vi "qrread.vi"() -> ()   [LabVIEW 2019]
uses:
  Global 1.vi
  <vilib>/vision/driver/NI_Vision_Acquisition_Software.lvlib
  <vilib>/userDefined/High Color/IMAQdx.ctl
  <vilib>/myRIO/Instrument Drivers/Utilities/Utilities.lvlib
  <vilib>/myRIO/Common/Instrument Driver Framework/myRIO v1.0/DIO/typedefs/DIO Channels Enum.ctl
  <vilib>/myRIO/Common/Instrument Driver Framework/myRIO v1.0/DIO/typedefs/DIO Channels List.ctl
  <vilib>/myRIO/Common/Instrument Driver Framework/Utilities/typedefs/Generic FPGA Reference.ctl
  <vilib>/myRIO/Common/Instrument Driver Framework/Utilities/typedefs/myRIO v1.0 Reference.ctl
  <vilib>/myRIO/Common/Instrument Driver Framework/Utilities/typedefs/Hardware Version Enum.ctl
  <vilib>/myRIO/Common/Instrument Driver Framework/Utilities/typedefs/myRIO Generic Hardware Reference.ctl
  <vilib>/myRIO/Instrument Drivers/Onboard IO/DIO/typedefs/DIO Reference.ctl
  <vilib>/myRIO/Instrument Drivers/Onboard IO/DIO/DIO.lvlib
  <vilib>/myRIO/Instrument Drivers/Onboard IO/DIO/vis/Write.vi
  <vilib>/userDefined/High Color/nirio_resource_hc.ctl
  <vilib>/myRIO/Common/Instrument Driver Framework/myRIO v1.0/DIO/vis/myRIO v1.1 Open DIO.vi
  <vilib>/myRIO/Instrument Drivers/Onboard IO/DIO/vis/myRIO DIO Open.xnode
  <vilib>/myRIO/Common/Instrument Driver Framework/Utilities/vis/Is FPGA Ref Available.vi
  <vilib>/myRIO/Express VI/Onboard Devices/LED/LED Express VI.xnode
  <vilib>/myRIO/Express VI/Onboard IO/DO/DO Express VI.xnode
  <vilib>/myRIO/Express VI/Onboard IO/DI/DI Express VI.xnode
  <vilib>/myRIO/Instrument Drivers/Onboard IO/DIO/vis/Read.vi
  <vilib>/vision/Instrument.llb/QR Code Model Type.ctl
  <vilib>/vision/Instrument.llb/QR Code Stream Mode Type.ctl
  <vilib>/vision/Instrument.llb/Data Matrix Polarity.ctl
  <vilib>/vision/Instrument.llb/Demodulation Mode.ctl
  <vilib>/vision/Instrument.llb/Cell Sample Size.ctl
  <vilib>/vision/Instrument.llb/Cell Filter Mode.ctl
  <vilib>/vision/Instrument.llb/QR Code Report.ctl
panel:
  out "Refnum out 4":T1(plugin-control)
  out "Refnum out 3":T1(plugin-control)
  in  "Error/Flow In":errorcluster
  out "Refnum out 2":T1(plugin-control)
  out "Refnum out":T1(plugin-control)
  out "t":i32
  out "Array":bool[](array[boolean])
  out "appended array":bool[](array[boolean])
  out "Found?":bool
  out "Bounding Box":cluster{"x":sgl, "y":sgl}[](array[cluster])
  out "QR Barcode Report (2D Barcode Reader 1)":T2={"Found?"=FALSE, "Data"="", "Bounding Box"=[], "Errors Corrected"=0, "Dimensions (Rows/Cols)"=0, "Version"=0, "QR Model"=3, "Stream Mode"=0, "Barcode Polarity"=-2, "Mirrored?"=FALSE, "Append Stream Position"=0, "Size of Append Stream"=0, "First EAN-128 ID"=0, "First Alternate Language ID"=0, "Append Stream ID"=0, "Minimum Edge Strength"=30, "Demodulation Mode"=-2, "Cell Sample Size"=-2, "Cell Filter Mode"=-2} {"Append Stream ID" format="%x"; "Cell Filter Mode" items=["Auto-detect"=-2, "Average"=0, "Median"=1, "Central Average"=2, "High Average"=3, "Low Average"=4, "Very High Average"=5, "Very Low Average"=6, "All Filters"=8]; "Cell Sample Size" items=["Auto-detect"=-2, "1x1"=1, "2x2"=2, "3x3"=3, "4x4"=4, "5x5"=5, "6x6"=6, "7x7"=7]; "Demodulation Mode" items=["Auto-detect"=-2, "Histogram"=0, "Local Contrast"=1, "Combination"=2, "All"=3]; "Barcode Polarity" items=["Auto-detect"=-2, "Black on White"=0, "White on Black"=1]; "Stream Mode" items=["Auto-detect", "Numeric", "AlphaNumeric", "Mixed", "Raw Bytes", "UCC/EAN-128 - In Tokens", "UCC/EAN-128 - In Data", "Extended Character Interpretation", "Kanji"]; "QR Model" items=["Auto Detect", "Micro", "Model 1", "Model 2"]; "Version" max=40 step=1}
  in  "Stop (F)":bool
  out "Image Out":T1(plugin-control)
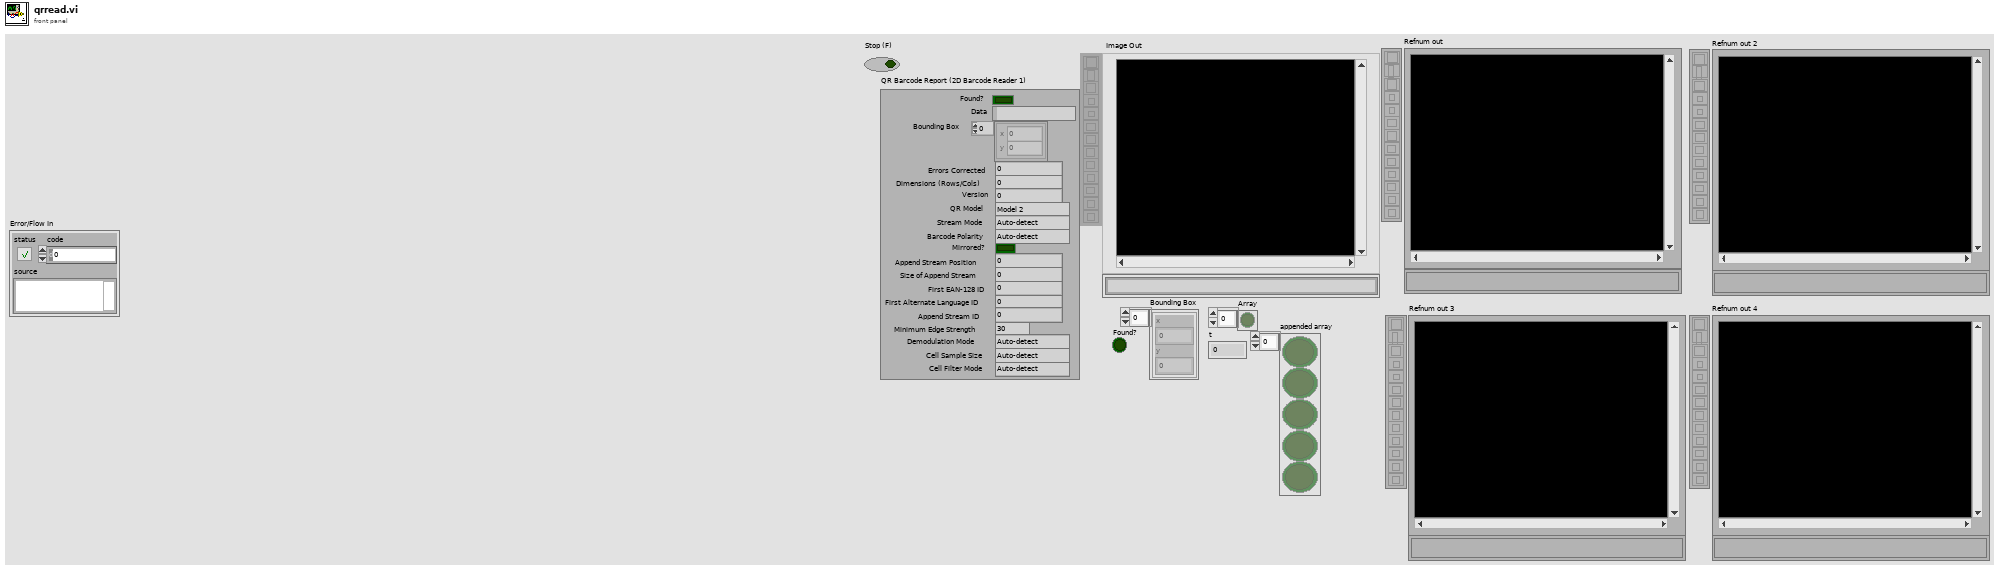
[diagram p1: front panel]
types:
  T1 = typedef "IMAQ Image.ctl" = refnum<image>
  T2 = typedef "QR Code Report.ctl" = cluster{"Found?":bool, "Data":string, "Bounding Box":cluster{"x":sgl, "y":sgl}[], "Errors Corrected":u32, "Dimensions (Rows/Cols)":u32, "Version":u32, "QR Model":T3, "Stream Mode":T4, "Barcode Polarity":T5, "Mirrored?":bool, "Append Stream Position":u32, "Size of Append Stream":u32, "First EAN-128 ID":i32, "First Alternate Language ID":i32, "Append Stream ID":u32, "Minimum Edge Strength":u32, "Demodulation Mode":T6, "Cell Sample Size":T7, "Cell Filter Mode":T8}
  T3 = typedef "QR Code Model Type.ctl" = i32
  T4 = typedef "QR Code Stream Mode Type.ctl" = i32
  T5 = typedef "Data Matrix Polarity.ctl" = i32
  T6 = typedef "Demodulation Mode.ctl" = i32
  T7 = typedef "Cell Sample Size.ctl" = i32
  T8 = typedef "Cell Filter Mode.ctl" = i32
  T9 = typedef "IMAQdx.ctl" = refnum<k21>
  T10 = typedef "DIO.lvlib/DIO Reference.ctl" = cluster{"myRIO Reference":T11, "DIO Channels List":T15}
  T11 = typedef "myRIO Generic Hardware Reference.ctl" = cluster{"myRIO Model":T12, "myRIO Hardware Reference":T13}
  T12 = typedef "Hardware Version Enum.ctl" = enum16{"Unknown", "myRIO-1900", "myRIO-1950", "roboRIO", "NI ELVIS RIO CM", "ELVIS III"}
  T13 = typedef "myRIO v1.0 Reference.ctl" = cluster{"Generic FPGA Reference":T14, "Allow multiple opens":bool}
  T14 = typedef "Generic FPGA Reference.ctl" = refnum<k20>
  T15 = typedef "DIO Channels List.ctl" = T16[]
  T16 = typedef "DIO Channels Enum.ctl" = enum16{"Not Connected", "C/DIO0", "C/DIO1", "C/DIO2", "C/DIO3", "C/DIO4", "C/DIO5", "C/DIO6", "C/DIO7", "A/DIO0", "A/DIO1", "A/DIO2", "A/DIO3", "A/DIO4", "A/DIO5", "A/DIO6", "A/DIO7", "A/DIO8", "A/DIO9", "A/DIO10", "A/DIO11", "A/DIO12", "A/DIO13", "A/DIO14", "A/DIO15", "A/DIO16", "A/DIO17", "A/DIO18", "A/DIO19", "B/DIO0", "B/DIO1", "B/DIO2", "B/DIO3", "B/DIO4", "B/DIO5", "B/DIO6", "B/DIO7", "B/DIO8", "B/DIO9", "B/DIO10", "B/DIO11", "B/DIO12", "B/DIO13", "B/DIO14", "B/DIO15", "B/DIO16", "B/DIO17", "B/DIO18", "B/DIO19", "LED0", "LED1", "LED2", "LED3", "Button0", "DIO/DIO0", "DIO/DIO1", "DIO/DIO2", "DIO/DIO3", "DIO/DIO4", "DIO/DIO5", "DIO/DIO6", "DIO/DIO7", "DIO/DIO8", "DIO/DIO9", "SPI/CS0", "SPI/CS1", "SPI/CS2", "SPI/CS3", "LED RADIO (Green)", "LED RADIO (Red)", "LED COMM (Green)", "LED COMM (Red)", "LED MODE (Green)", "LED MODE (Red)"}
  T17 = typedef "nirio_resource_hc.ctl" = tag
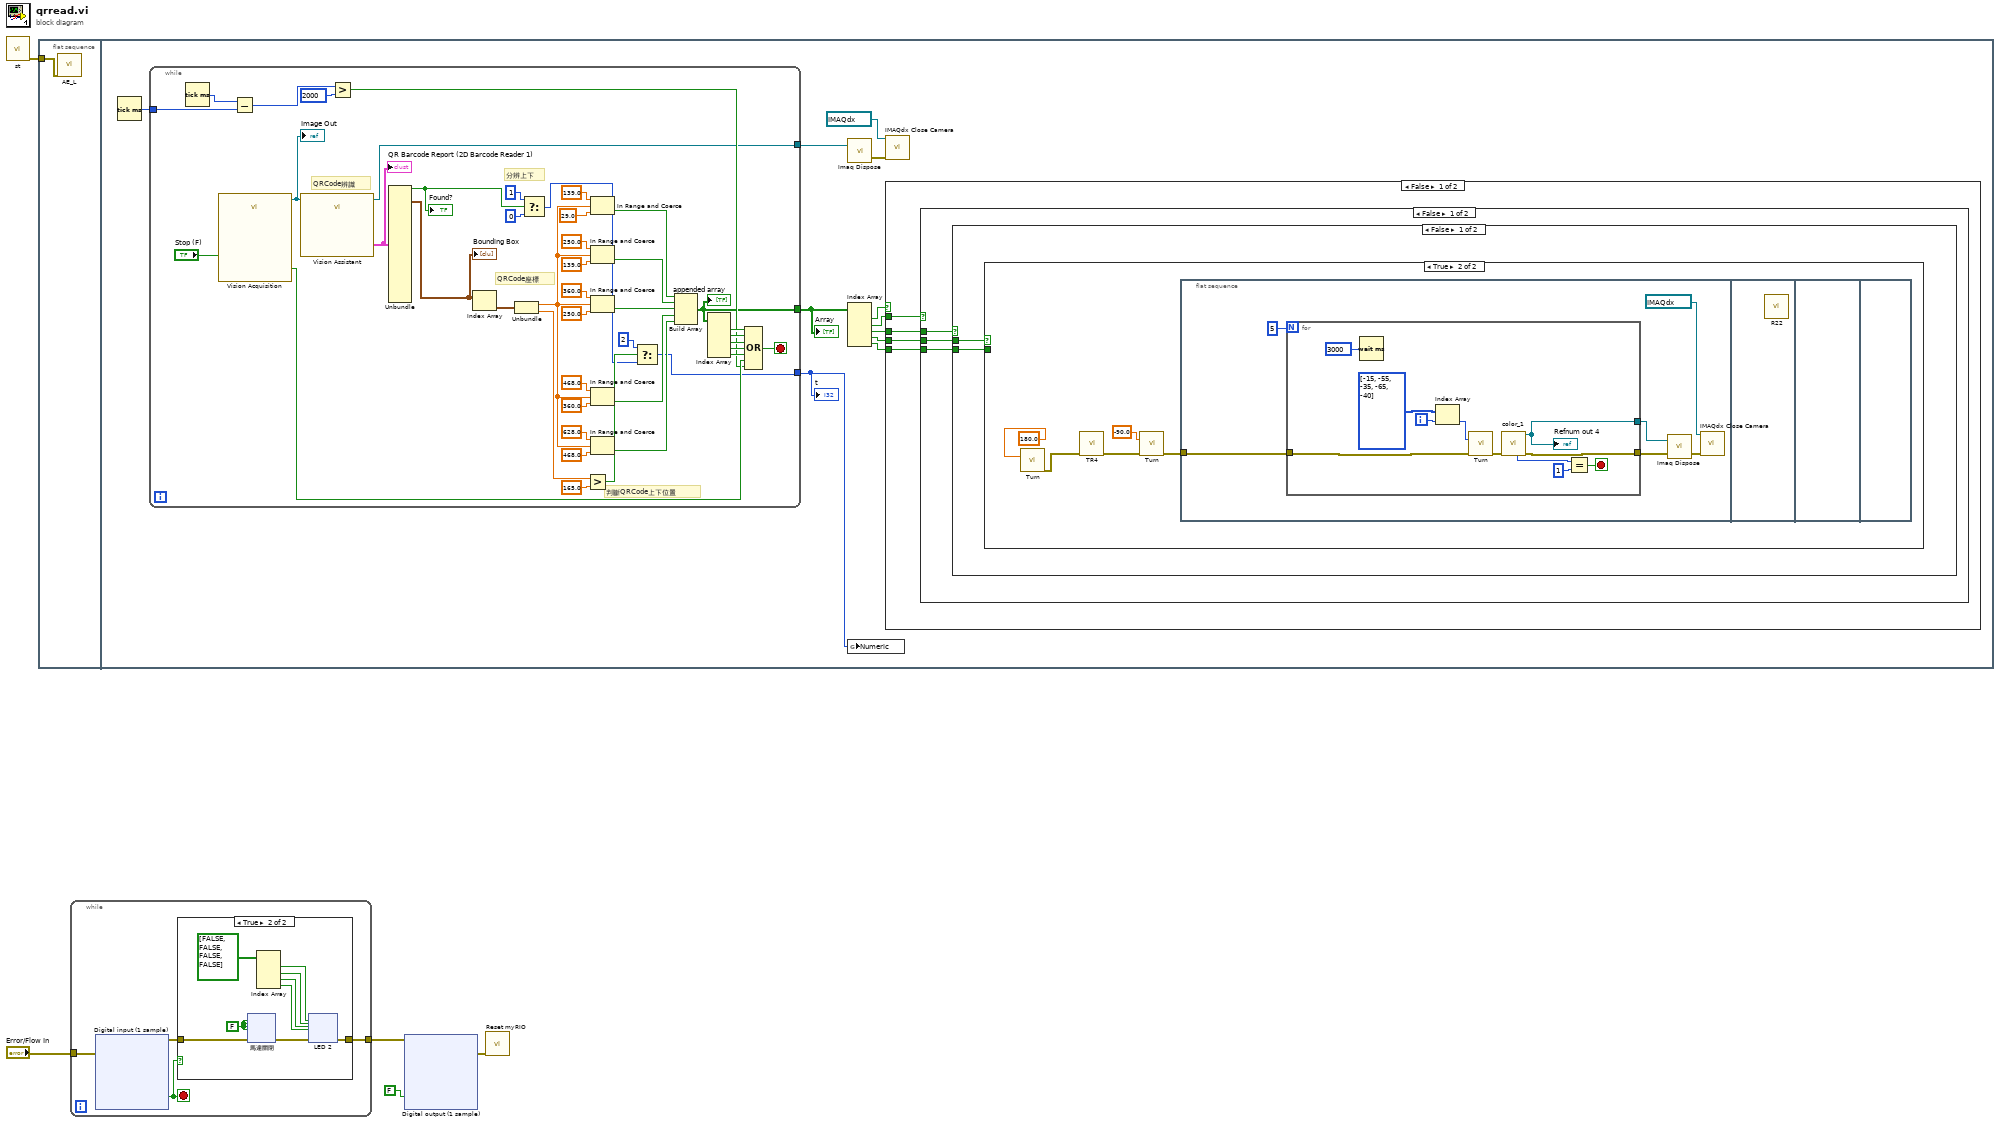
[diagram p0: block diagram]
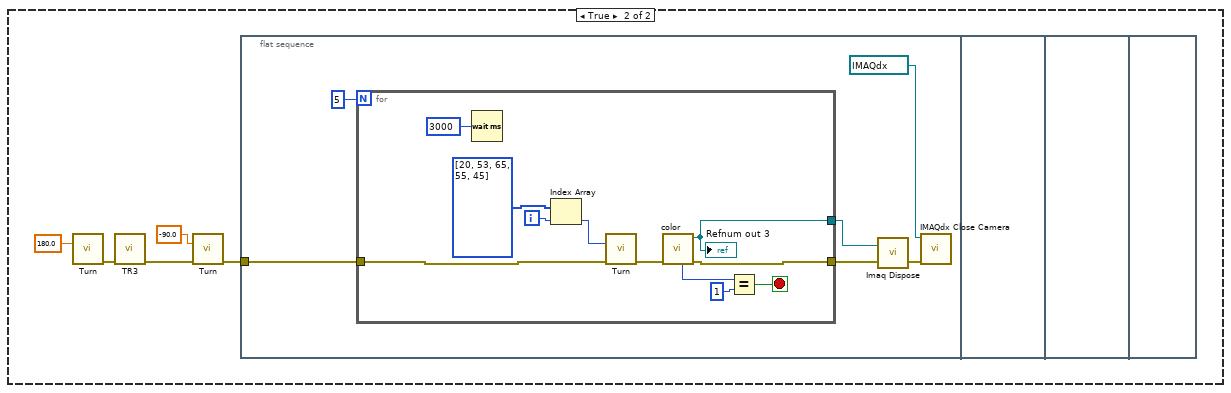
[diagram p5: hidden frame]
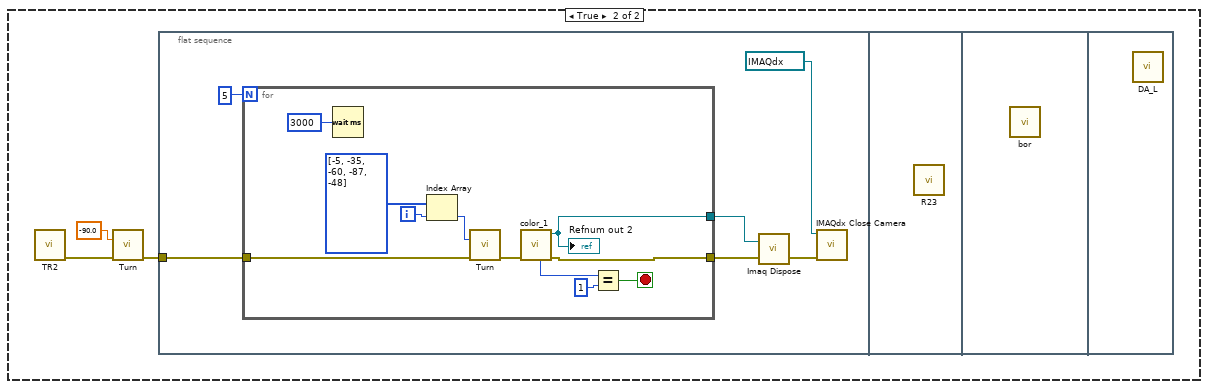
[diagram p6: hidden frame]
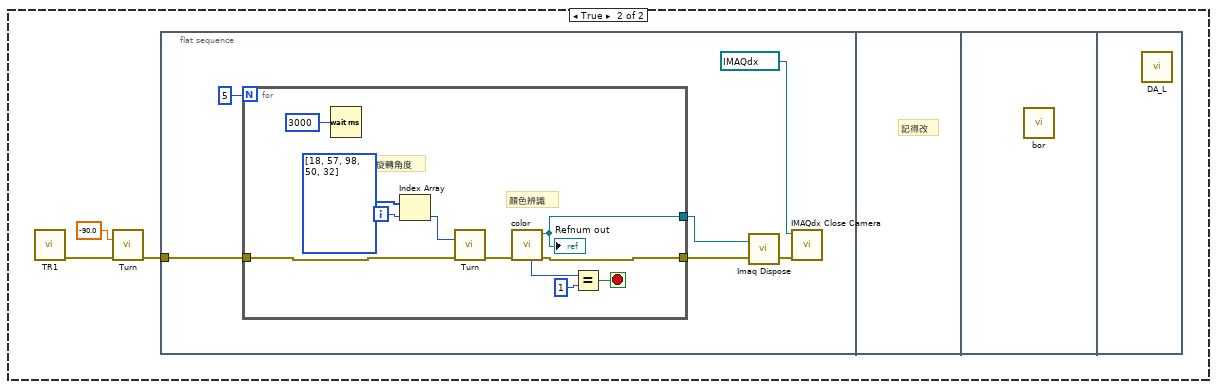
[diagram p7: hidden frame]
diagram:
  n1 = call "st.vi"() -> ("Error/Flow Out"=w5:errorcluster)  [unwired: 11 in]
  n2 = flat-sequence {
    tunnel: w5 -> [w6]
    frame #0 {
      n3 = call "AE_L.vi"("error in (no error)"=w6) -> ()  [unwired: 10 in, 1 out]
    }
    frame #1 {
      n4 = Tick Count (ms)() -> (millisecond timer value=w17:u32)
      n5 = while {
        tunnel: w17 -> [w135]
        tunnel: [w124] -> w16
        tunnel: [w115] -> w10
        tunnel: [w112] -> w9
        stop <- w125 stop-if-true
        # "分辨上下"
        # "QRCode辨識"
        # "判斷QRCode上下位置"
        # "QRCode座標"
        n6 = Tick Count (ms)() -> (millisecond timer value=w136:u32)
        n7 = call "Vision Acquisition"("Stop (F)"="Stop (F)") -> ("Image Out"=w114:T1, "Stopped"=w127:bool)  [unwired: 24 in, 1 out]
        "Image Out" <- w114
        n8 = Subtract(x=w136, y=w135) -> (x-y=w134:u32)
        n9 = call "Vision Assistant"("Image In"=w114) -> ("Image Out"=w112:T1, "QR Barcode Report (2D Barcode Reader 1)"=w113:T2)  [unwired: 24 in, 1 out]
        "QR Barcode Report (2D Barcode Reader 1)" <- w113
        n10 = Greater?(x=w134, y=u32 2000) -> (0:w126:bool)
        n11 = Unbundle(w113) -> ("Found?"=w120:bool, "Bounding Box"=w154:cluster{"x":sgl, "y":sgl}[])  [unwired: 17 out]
        "Bounding Box" <- w154
        "Found?" <- w120
        n12 = Index Array(array=w154) -> (element=w143:cluster{"x":sgl, "y":sgl})  [unwired: 1 in]
        n13 = Unbundle(w143) -> ("x"=w142:sgl, "y"=w123:sgl)
        n14 = Select(t=1, s=w120, f=0) -> (s? t:f=w117:i32)
        n15 = Greater?(x=w123, y=sgl 165.0) -> (0:w121:bool)
        n16 = In Range and Coerce(upper limit=139.0, x=w142, lower limit=29.0) -> (In Range?=w141:bool)  [unwired: 1 out]
        n17 = In Range and Coerce(upper limit=250.0, x=w142, lower limit=139.0) -> (In Range?=w140:bool)  [unwired: 1 out]
        n18 = In Range and Coerce(upper limit=360.0, x=w142, lower limit=250.0) -> (In Range?=w139:bool)  [unwired: 1 out]
        n19 = In Range and Coerce(upper limit=468.0, x=w142, lower limit=360.0) -> (In Range?=w138:bool)  [unwired: 1 out]
        n20 = In Range and Coerce(upper limit=628.0, x=w142, lower limit=468.0) -> (In Range?=w137:bool)  [unwired: 1 out]
        n21 = Select(t=2, s=w121, f=w117) -> (s? t:f=w115:i32)
        n22 = Build Array(w141, w140, w139, w138, w137) -> (w124:bool[])
        "appended array" <- w124
        n23 = Index Array(array=w124) -> (element #1=w132:bool, element #2=w131:bool, element #3=w130:bool, element #4=w129:bool, element #5=w128:bool)  [unwired: 5 in]
        n24 = Compound Arithmetic op=OR(w132, w131, w130, w129, w128, w127, w126) -> (w125:bool)
      }
      "Array" <- w16
      "t" <- w10
      n25 = call "Imaq Dispose"("Image"=w9) -> ("error out"=w8:errorcluster)  [unwired: 5 in]
      n26 = Index Array(array=w16) -> (element #1=w15:bool, element #2=w14:bool, element #3=w13:bool, element #4=w12:bool, element #5=w11:bool)  [unwired: 5 in]
      n27 = global write "Global 1.vi" "Numeric"(w10) -> ()
      n28 = call <vilib>:"IMAQdx Close Camera.vi"("error in"=w8, "Session In"=T9 "cam0") -> ()  [unwired: 9 in, 1 out]
      n29 = case shown="False" w15 {
        tunnel: w14 -> [w21 _]
        tunnel: w13 -> [w20 _]
        tunnel: w12 -> [w19 _]
        tunnel: w11 -> [w18 _]
        frame False {
          n30 = case shown="False" w21 {
            tunnel: w20 -> [w24 _]
            tunnel: w19 -> [w23 _]
            tunnel: w18 -> [w22 _]
            frame False {
              n31 = case shown="False" w24 {
                tunnel: w23 -> [w26 _]
                tunnel: w22 -> [w25 _]
                frame False {
                  n32 = case shown="True" w26 {
                    tunnel: w25 -> [w27 _]
                    frame False {
                      n33 = case shown="True" w27 {
                        frame False {
                        }
                        frame True {
                        }
                      }
                    }
                    frame True {
                      n34 = call "Turn.vi"("角度"=180.0) -> ("error out"=w28:errorcluster)  [unwired: 14 in]
                      n35 = call "TR4.vi"("error in (no error)"=w28) -> ("error out"=w29:errorcluster)  [unwired: 10 in]
                      n36 = call "Turn.vi"("角度"=-90.0, "error in (no error)"=w29) -> ("error out"=w31:errorcluster)  [unwired: 13 in]
                      n37 = flat-sequence {
                        tunnel: w31 -> [w37]
                        frame #0 {
                          n38 = for {
                            N: 5 -> [_]
                            tunnel: w37 -> [w42]
                            tunnel: [w40] -> w33
                            tunnel: [w39] -> w35
                            i -> [w45]
                            stop <- w46 stop-if-true
                            n39 = Wait (ms)(milliseconds to wait=u32 3000) -> ()  [unwired: 1 out]
                            n40 = Index Array(array=i32[] [-15, -55, -35, -65, -40], index=w45) -> (element=w44:i32)
                            n41 = call "Turn.vi"("角度"=w44, "error in (no error)"=w42) -> ("error out"=w41:errorcluster)  [unwired: 13 in]
                            n42 = call "color_1.vi"("error in"=w41) -> ("error out"=w40:errorcluster, "Refnum out"=w39:T1, "yellow"=w43:i32)  [unwired: 3 in, 5 out]
                            "Refnum out 4" <- w39
                            n43 = Equal?(x=w43, y=1) -> (x = y?=w46:bool)
                          }
                          n44 = call "Imaq Dispose"("Image"=w35, "error in (no error)"=w33) -> ("error out"=w34:errorcluster)  [unwired: 4 in]
                          n45 = call <vilib>:"IMAQdx Close Camera.vi"("error in"=w34, "Session In"=T9 "cam0") -> ()  [unwired: 9 in, 1 out]
                        }
                        frame #1 {
                          n46 = call "R22.vi"() -> ()  [unwired: 12 in]
                        }
                        frame #2 {
                        }
                        frame #3 {
                        }
                      }
                    }
                  }
                }
                frame True {
                  n47 = call "Turn.vi"("角度"=180.0) -> ("error out"=w54:errorcluster)  [unwired: 14 in]
                  n48 = call "TR3.vi"("error in (no error) 2"=w54) -> ("error out 2"=w50:errorcluster)  [unwired: 10 in]
                  n49 = call "Turn.vi"("角度"=-90.0, "error in (no error)"=w50) -> ("error out"=w52:errorcluster)  [unwired: 13 in]
                  n50 = flat-sequence {
                    tunnel: w52 -> [w59]
                    frame #0 {
                      n51 = for {
                        N: 5 -> [_]
                        tunnel: w59 -> [w65]
                        tunnel: [w63] -> w55
                        tunnel: [w61] -> w57
                        i -> [w67]
                        stop <- w68 stop-if-true
                        n52 = Wait (ms)(milliseconds to wait=u32 3000) -> ()  [unwired: 1 out]
                        n53 = Index Array(array=i32[] [20, 53, 65, 55, 45], index=w67) -> (element=w66:i32)
                        n54 = call "Turn.vi"("角度"=w66, "error in (no error)"=w65) -> ("error out"=w64:errorcluster)  [unwired: 13 in]
                        n55 = call "color.vi"("error in"=w64) -> ("error out"=w63:errorcluster, "Refnum out"=w61:T1, "yellow"=w62:i32)  [unwired: 3 in, 5 out]
                        "Refnum out 3" <- w61
                        n56 = Equal?(x=w62, y=1) -> (x = y?=w68:bool)
                      }
                      n57 = call "Imaq Dispose"("Image"=w57, "error in (no error)"=w55) -> ("error out"=w56:errorcluster)  [unwired: 4 in]
                      n58 = call <vilib>:"IMAQdx Close Camera.vi"("error in"=w56, "Session In"=T9 "cam0") -> ()  [unwired: 9 in, 1 out]
                    }
                    frame #1 {
                    }
                    frame #2 {
                    }
                    frame #3 {
                    }
                  }
                }
              }
            }
            frame True {
              n59 = call "TR2.vi"() -> ("error out"=w73:errorcluster)  [unwired: 11 in]
              n60 = call "Turn.vi"("角度"=-90.0, "error in (no error)"=w73) -> ("error out"=w74:errorcluster)  [unwired: 13 in]
              n61 = flat-sequence {
                tunnel: w74 -> [w79]
                frame #0 {
                  n62 = for {
                    N: 5 -> [_]
                    tunnel: w79 -> [w84]
                    tunnel: [w82] -> w75
                    tunnel: [w81] -> w77
                    i -> [w87]
                    stop <- w88 stop-if-true
                    n63 = Wait (ms)(milliseconds to wait=u32 3000) -> ()  [unwired: 1 out]
                    n64 = Index Array(array=i32[] [-5, -35, -60, -87, -48], index=w87) -> (element=w86:i32)
                    n65 = call "Turn.vi"("角度"=w86, "error in (no error)"=w84) -> ("error out"=w83:errorcluster)  [unwired: 13 in]
                    n66 = call "color_1.vi"("error in"=w83) -> ("error out"=w82:errorcluster, "Refnum out"=w81:T1, "yellow"=w85:i32)  [unwired: 3 in, 5 out]
                    "Refnum out 2" <- w81
                    n67 = Equal?(x=w85, y=1) -> (x = y?=w88:bool)
                  }
                  n68 = call "Imaq Dispose"("Image"=w77, "error in (no error)"=w75) -> ("error out"=w76:errorcluster)  [unwired: 4 in]
                  n69 = call <vilib>:"IMAQdx Close Camera.vi"("error in"=w76, "Session In"=T9 "cam0") -> ()  [unwired: 9 in, 1 out]
                }
                frame #1 {
                  n70 = call "R23.vi"() -> ()  [unwired: 12 in]
                }
                frame #2 {
                  n71 = call "bor.vi"() -> ()  [unwired: 12 in]
                }
                frame #3 {
                  n72 = call "DA_L.vi"() -> ()  [unwired: 11 in, 1 out]
                }
              }
            }
          }
        }
        frame True {
          n73 = call "TR1.vi"() -> ("error out"=w94:errorcluster)  [unwired: 11 in]
          n74 = call "Turn.vi"("角度"=-90.0, "error in (no error)"=w94) -> ("error out"=w92:errorcluster)  [unwired: 13 in]
          n75 = flat-sequence {
            tunnel: w92 -> [w99]
            frame #0 {
              n76 = for {
                N: 5 -> [_]
                tunnel: w99 -> [w105]
                tunnel: [w103] -> w95
                tunnel: [w102] -> w97
                i -> [w107]
                stop <- w108 stop-if-true
                # "旋轉角度"
                # "顏色辨識"
                n77 = Wait (ms)(milliseconds to wait=u32 3000) -> ()  [unwired: 1 out]
                n78 = Index Array(array=i32[] [18, 57, 98, 50, 32], index=w107) -> (element=w106:i32)
                n79 = call "Turn.vi"("角度"=w106, "error in (no error)"=w105) -> ("error out"=w104:errorcluster)  [unwired: 13 in]
                n80 = call "color.vi"("error in"=w104) -> ("error out"=w103:errorcluster, "Refnum out"=w102:T1, "yellow"=w101:i32)  [unwired: 3 in, 5 out]
                "Refnum out" <- w102
                n81 = Equal?(x=w101, y=1) -> (x = y?=w108:bool)
              }
              n82 = call "Imaq Dispose"("Image"=w97, "error in (no error)"=w95) -> ("error out"=w96:errorcluster)  [unwired: 4 in]
              n83 = call <vilib>:"IMAQdx Close Camera.vi"("error in"=w96, "Session In"=T9 "cam0") -> ()  [unwired: 9 in, 1 out]
            }
            frame #1 {
              # "記得改"
            }
            frame #2 {
              n84 = call "bor.vi"() -> ()  [unwired: 12 in]
            }
            frame #3 {
              n85 = call "DA_L.vi"() -> ()  [unwired: 11 in, 1 out]
            }
          }
        }
      }
    }
  }
  n86 = while {
    tunnel: "Error/Flow In" -> [w158]
    tunnel: [w157] -> w3
    stop <- w156 stop-if-true
    n87 = xnode "Digital input (1 sample)"("error in (no error)"=w158) -> ("C/DIO5 (DIO5)"=w156:bool, "error out"=w159:errorcluster)
    n88 = case shown="True" w156 {
      tunnel: w159 -> [w195 w198]
      tunnel: [w195 w196] -> w157
      frame False {
      }
      frame True {
        w200 = FALSE ("A/DIO1 (Pin 13)")
        n89 = xnode "馬達關閉"("error in (no error)"=w198, "A/DIO1 (Pin 13)"=w200, "A/DIO4 (Pin 19)"=w200, "B/DIO1 (Pin 13)"=w200, "B/DIO4 (Pin 19)"=w200) -> ("error out"=w197:errorcluster)
        n90 = Index Array(array=bool[] [FALSE, FALSE, FALSE, FALSE]) -> (element #1=w204:bool, element #2=w203:bool, element #3=w202:bool, element #4=w201:bool)  [unwired: 4 in]
        n91 = xnode "LED 2"("error in (no error)"=w197, "LED0"=w204, "LED1"=w203, "LED2"=w202, "LED3"=w201) -> ("error out"=w196:errorcluster)
      }
    }
  }
  n92 = xnode "Digital output (1 sample)"("C/DIO1 (DIO1)"=FALSE, "error in (no error)"=w3) -> ("error out"=w2:errorcluster)
  n93 = call <vilib>:"Reset myRIO.vi"("error in (no error)"=w2) -> ()  [unwired: 10 in, 1 out]
